vi "Swap.vi"(9 "Y":i32, 10 "X":i32, 11 "Unswapped Array":dbl[](array[numeric])) -> (3 "Swapped Array":dbl[](array[numeric]))   [LabVIEW 2015]
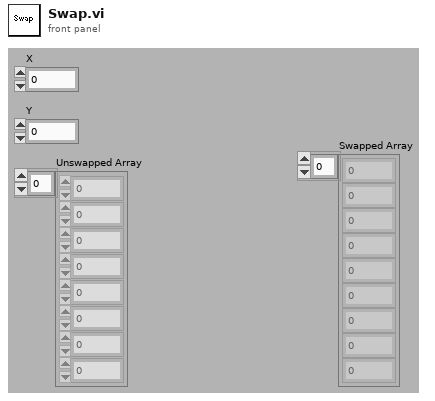
[diagram p1: front panel]
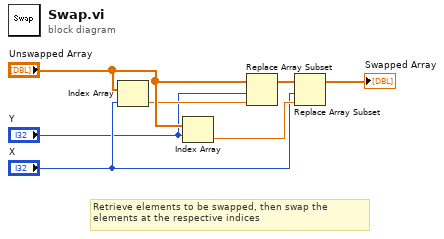
[diagram p0: block diagram]
diagram:
  # "Retrieve elements to be swapped, then swap the \nelements at the respective indices"
  n1 = Index Array(array="Unswapped Array", index="X") -> (element=w6:dbl)
  n2 = Index Array(array="Unswapped Array", index="Y") -> (element=w5:dbl)
  n3 = Replace Array Subset(array="Unswapped Array", new element=w6, index="Y") -> (w1:dbl[])
  n4 = Replace Array Subset(array=w1, new element=w5, index="X") -> (→"Swapped Array":dbl[])
